vi "AO add remove elements.vi"(1 "NewVal in":T1 {"f (Hz)" min=0.001 max=10000.0 format="%.3g"; "Phase (°)" format="%.3g"; "DC (V)" format="%.3p"; "Amp (V)" min=0.0 max=10.0 format="%.3p"}) -> (0 "NewVal out":T1 {"f (Hz)" min=0.001 max=10000.0 format="%.3g"; "Phase (°)" format="%.3g"; "DC (V)" format="%.3p"; "Amp (V)" min=0.0 max=10.0 format="%.3p"})   [LabVIEW 2016, in "Instrument.Lockin.lvclass"]
uses:
  Instrument.Lockin.lvclass
  LockinDAQ/Typedefs/AO-cluster.ctl
  LockinDAQ/Typedefs/Function-enum.ctl
  LockinDAQ/LockinDAQ.lvclass
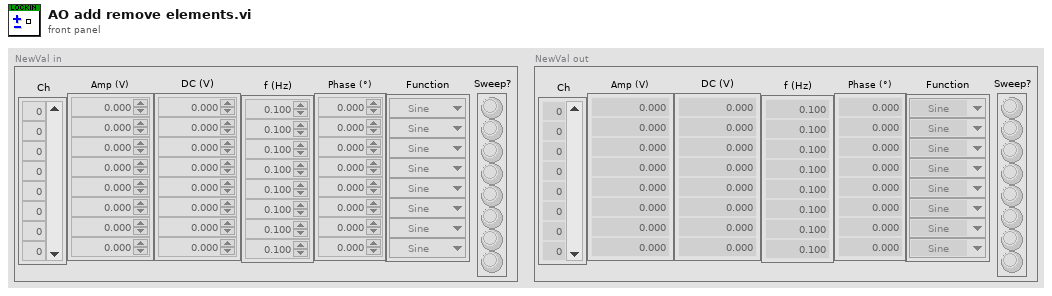
[diagram p1: front panel]
types:
  T1 = typedef "LockinDAQ.lvclass/AO-cluster.ctl" = cluster{"Ch":i32[], "Amp (V)":dbl[], "DC (V)":dbl[], "f (Hz)":dbl[], "Phase (°)":dbl[], "Function":T2[], "Sweep?":bool[]}
  T2 = typedef "LockinDAQ.lvclass/Function-enum.ctl" = enum16{"Sine", "Triangle", "Square", "Sawtooth"}
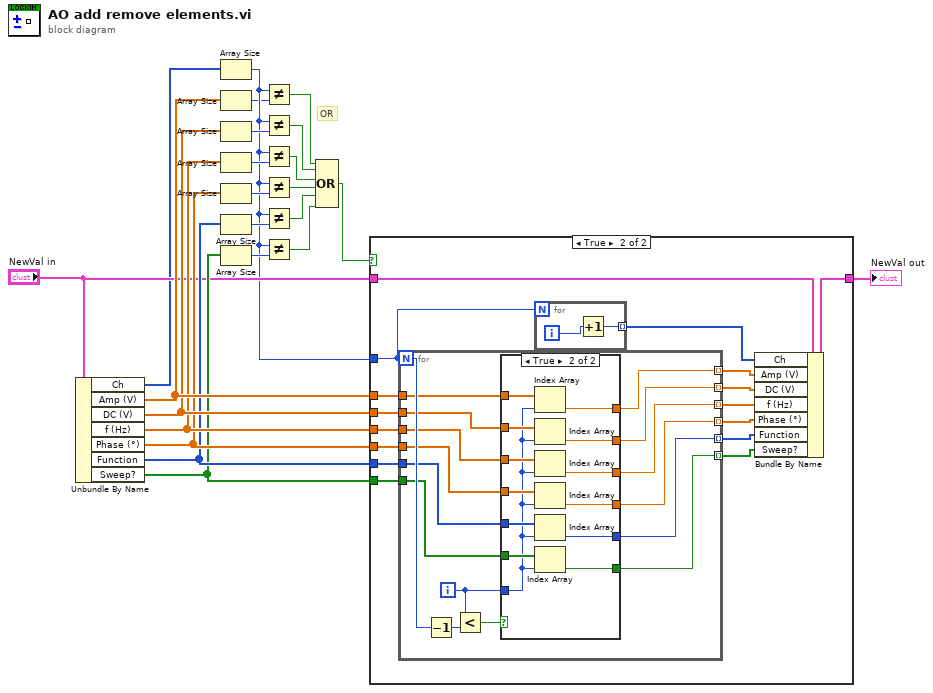
[diagram p0: block diagram]
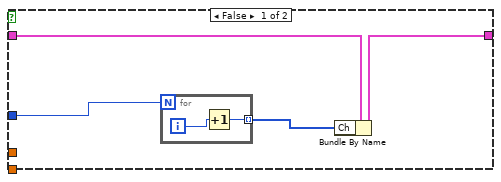
[diagram p2: hidden frame]
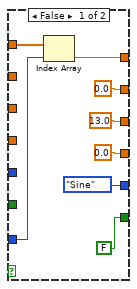
[diagram p3: hidden frame]
diagram:
  # "OR"
  n1 = Unbundle By Name("NewVal in") -> ("Ch"=w9:i32[], "Amp (V)"=w16:dbl[], "DC (V)"=w15:dbl[], "f (Hz)"=w14:dbl[], "Phase (°)"=w13:dbl[], "Function"=w12:T2[], "Sweep?"=w11:bool[])
  n2 = Array Size(array=w9) -> (size(s)=w8:i32)
  n3 = Array Size(array=w16) -> (size(s)=w7:i32)
  n4 = Array Size(array=w15) -> (size(s)=w22:i32)
  n5 = Array Size(array=w14) -> (size(s)=w21:i32)
  n6 = Array Size(array=w13) -> (size(s)=w20:i32)
  n7 = Array Size(array=w12) -> (size(s)=w19:i32)
  n8 = Array Size(array=w11) -> (size(s)=w18:i32)
  n9 = Not Equal?(x=w8, y=w7) -> (x != y?=w1:bool)
  n10 = Not Equal?(x=w8, y=w22) -> (x != y?=w2:bool)
  n11 = Not Equal?(x=w8, y=w21) -> (x != y?=w3:bool)
  n12 = Not Equal?(x=w8, y=w20) -> (x != y?=w4:bool)
  n13 = Not Equal?(x=w8, y=w19) -> (x != y?=w5:bool)
  n14 = Not Equal?(x=w8, y=w18) -> (x != y?=w6:bool)
  n15 = Compound Arithmetic op=OR(w1, w2, w3, w4, w5, w6) -> (w17:bool)
  n16 = case shown="True" w17 {
    tunnel: [w24 w32] -> w23
    tunnel: "NewVal in" -> [w25 w45]
    tunnel: w8 -> [w27 w31]
    tunnel: w16 -> [_ w41]
    tunnel: w15 -> [_ w40]
    tunnel: w14 -> [_ w39]
    tunnel: w13 -> [_ w38]
    tunnel: w12 -> [_ w37]
    tunnel: w11 -> [_ w36]
    frame False {
      n17 = for {
        N: w27 -> [_]
        tunnel: [w28] -> w26 mode=indexing
        i -> [w29]
        n18 = Increment(x=w29) -> (x+1=w28:i32)
      }
      n19 = Bundle By Name(cluster=w25, "Ch"=w26) -> (w24:T1)
    }
    frame True {
      n20 = for {
        N: w31 -> [w63]
        tunnel: [w58] -> w34 mode=indexing
        tunnel: [w62] -> w44 mode=indexing
        tunnel: [w61] -> w43 mode=indexing
        tunnel: [w57] -> w42 mode=indexing
        tunnel: w41 -> [w50]
        tunnel: w40 -> [w54]
        tunnel: w39 -> [w51]
        tunnel: w38 -> [w49]
        tunnel: w37 -> [w55]
        tunnel: w36 -> [w56]
        tunnel: [w60] -> w35 mode=indexing
        tunnel: [w59] -> w33 mode=indexing
        i -> [w48]
        n21 = Decrement(x=w63) -> (x-1=w52:i32)
        n22 = Less?(x=w48, y=w52) -> (x < y?=w53:bool)
        n23 = case shown="True" w53 {
          tunnel: w50 -> [w71 w84]
          tunnel: w48 -> [w70 w72]
          tunnel: [w69 w73] -> w62
          tunnel: [0.0 ("AO DC") w83] -> w61
          tunnel: [13.0 ("AO f") w82] -> w60
          tunnel: [0.0 ("AO phi") w81] -> w59
          tunnel: [Function-enum."Sine" ("Signal Type") w80] -> w58
          tunnel: [FALSE ("Boolean") w79] -> w57
          tunnel: w56 -> [_ w78]
          tunnel: w49 -> [_ w77]
          tunnel: w55 -> [_ w76]
          tunnel: w51 -> [_ w75]
          tunnel: w54 -> [_ w74]
          frame False {
            n24 = Index Array(array=w71, index=w70) -> (element=w69:dbl)
          }
          frame True {
            n25 = Index Array(array=w84, index=w72) -> (element=w73:dbl)
            n26 = Index Array(array=w74, index=w72) -> (element=w83:dbl)
            n27 = Index Array(array=w75, index=w72) -> (element=w82:dbl)
            n28 = Index Array(array=w77, index=w72) -> (element=w81:dbl)
            n29 = Index Array(array=w76, index=w72) -> (element=w80:T2)
            n30 = Index Array(array=w78, index=w72) -> (element=w79:bool)
          }
        }
      }
      n31 = for {
        N: w31 -> [_]
        tunnel: [w46] -> w30 mode=indexing
        i -> [w47]
        n32 = Increment(x=w47) -> (x+1=w46:i32)
      }
      n33 = Bundle By Name(cluster=w45, "Ch"=w30, "Amp (V)"=w44, "DC (V)"=w43, "f (Hz)"=w35, "Phase (°)"=w33, "Function"=w34, "Sweep?"=w42) -> (w32:T1)
    }
  }
  "NewVal out" <- w23
